vi "Create.vi"(8 "error in (no error)":errorcluster, 10 "Log Reference":refnum<vi>) -> (0 "error out":errorcluster, 3 "String Indicator Logger":refnum<class "String Indicator Logger.lvclass">)   [LabVIEW 2020, in "String Indicator Logger.lvclass"]
uses:
  String Indicator Logger.lvclass
  String Indicator Logger.lvclass/String Indicator Logger.ctl
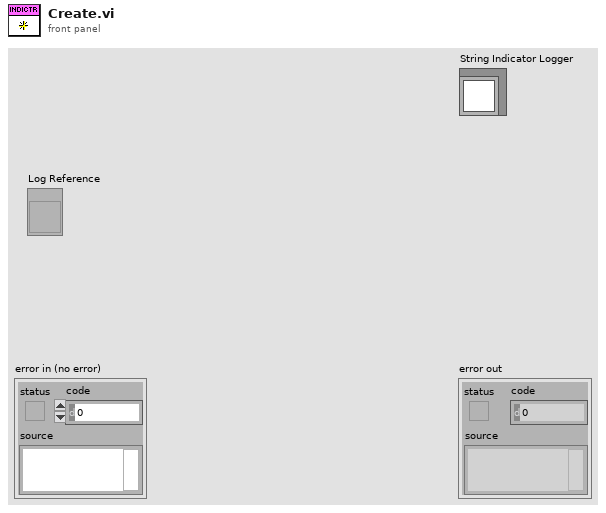
[diagram p1: front panel]
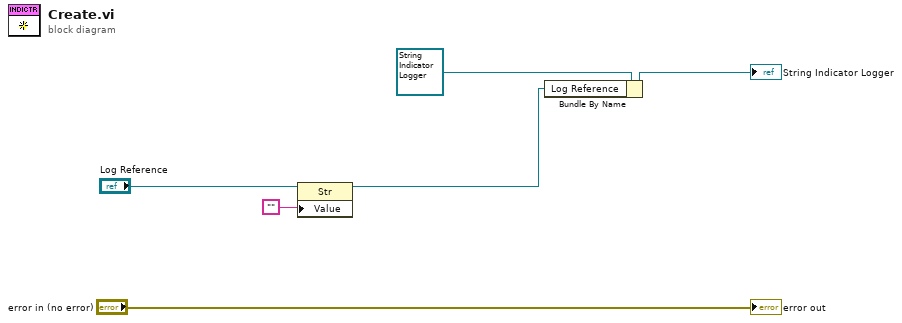
[diagram p0: block diagram]
diagram:
  n1 = property class="Str"(reference="Log Reference", "Value"="") -> (reference out=w2:refnum<vi>)  [unwired: 1 in, 1 out]
  n2 = Bundle By Name(cluster=refnum<class "String Indicator Logger.lvclass"> refnum ("String Indicator Logger"), "Log Reference"=w2) -> (→"String Indicator Logger":refnum<class "String Indicator Logger.lvclass">)
  "error out" <- "error in (no error)"
